vi "PropertyDelete.vi"(0 "Data":T1, 5 "error in":errorcluster) -> (14 "Data 2":T1, 19 "error out":errorcluster)   [LabVIEW 2017]
doc: "<B>This VI is used for delecte a property from the Caps file.</B>"
uses:
  Ctrl/compond commands.ctl
  Ctrl/Property.ctl
  Ctrl/PhysicalChannel.ctl
  Ctrl/Bitfield.ctl
  Ctrl/Register.ctl
  Ctrl/ScaleType.ctl
  Ctrl/Scale.ctl
  Ctrl/EnumValue.ctl
  Ctrl/Enum.ctl
  Ctrl/Caps.ctl
  Ctrl/Data.ctl
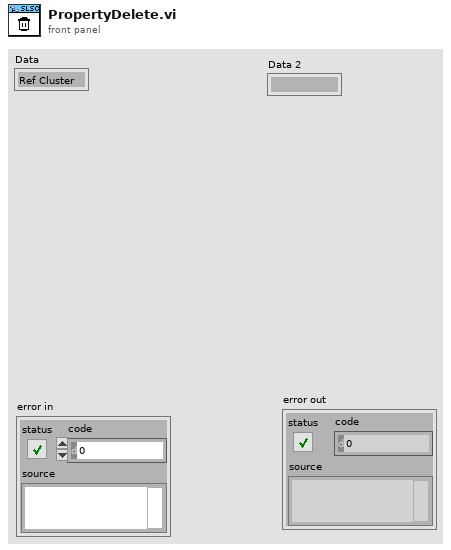
[diagram p1: front panel]
types:
  T1 = typedef "Data.ctl" = cluster{"Ref Cluster":cluster{"String":refnum<vi>, "U8":refnum<vi>, "I8":refnum<vi>, "U32":refnum<vi>, "I32":refnum<vi>, "U64":refnum<vi>, "I64":refnum<vi>, "Ring":refnum<vi>, "DBL":refnum<vi>, "Add":refnum<vi>, "Remove":refnum<vi>, "Property tree":refnum<vi>}, "JSON Text":string, "Original JSON Text":string, "Caps":T2, "SLSC Output Tree":cluster{"Left Cell String":string, "Child Text":string[], "Child Tag":string, "Item Indent":i32, "Child Only?":bool, "Glyph Index":i32, "offline value":variant}[], "Ref Index and Control Type":cluster{"index":i32, "Datatype":string}, "Selected Type and name":cluster{"Selected Type":enum16{"Property", "Physical Channel"}, "Selected Property Name":string}, "Update whole Tree?":bool}
  T2 = typedef "Caps.ctl" = cluster{"properties":T3[], "physical channels":T4[], "registers":T5[], "scales":T7[], "enums":T9[], "productName":string}
  T3 = typedef "Property.ctl" = cluster{"name":string, "bitfield":string, "value":variant, "dataType":string, "min":variant, "max":variant, "scale":string, "access":string}
  T4 = typedef "PhysicalChannel.ctl" = cluster{"name":string, "properties":T3[]}
  T5 = typedef "Register.ctl" = cluster{"name":string, "address":i32, "size":i32, "bitfields":T6[], "initialValue":variant, "connectedProperties":string[]}
  T6 = typedef "Bitfield.ctl" = cluster{"name":string, "offset":i32, "size":i32, "signed":bool}
  T7 = typedef "Scale.ctl" = cluster{"name":string, "type":T8, "params":variant}
  T8 = typedef "ScaleType.ctl" = enum16{"NoScale", "Table", "Polynomial", "Linear"}
  T9 = typedef "Enum.ctl" = cluster{"name":string, "values":T10[]}
  T10 = typedef "EnumValue.ctl" = cluster{"name":string, "value":i32}
  T11 = typedef "compond commands.ctl" = enum16{"Get Property Array", "Get Physical Channel Property Array", "Get the Selected Position", "Get Property and Physical Channel Name", "Get Type and Value", "Make and Set a new Property", "Modify the Value", "Delete a Property"}
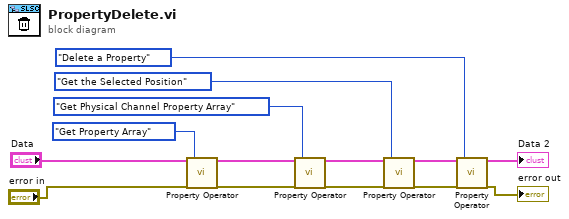
[diagram p0: block diagram]
diagram:
  n1 = call "Property Operator.vi"("Data"="Data", "error in"="error in", "Command"=compond_commands."Get Property Array") -> ("Data 2"=w13:T1, "error out"=w10:errorcluster)  [unwired: 13 in, 2 out]
  n2 = call "Property Operator.vi"("Data"=w13, "error in"=w10, "Command"=compond_commands."Get Physical Channel Property Array") -> ("Data 2"=w12:T1, "error out"=w9:errorcluster)  [unwired: 13 in, 2 out]
  n3 = call "Property Operator.vi"("Data"=w12, "error in"=w9, "Command"=compond_commands."Get the Selected Position") -> ("Data 2"=w6:T1, "error out"=w5:errorcluster)  [unwired: 13 in, 2 out]
  n4 = call "Property Operator.vi"("Data"=w6, "error in"=w5, "Command"=compond_commands."Delete a Property") -> ("Data 2"=→"Data 2":T1, "error out"=→"error out":errorcluster)  [unwired: 13 in, 2 out]
